vi "Write.vi"(10 "error in (no error)":errorcluster, 11 "Process_REF":string="Temperature") -> (0 "error out":errorcluster)   [LabVIEW 2018]
uses:
  <vilib>/DAQmx/write.llb/DAQmx Write (Digital Bool 1Line 1Point).vi
  <vilib>/DAQmx/create/channels.llb/DAQmx Create Channel (DO-Digital Output).vi
  <vilib>/DAQmx/miscellaneous.llb/DAQmx Fill In Error Info.vi
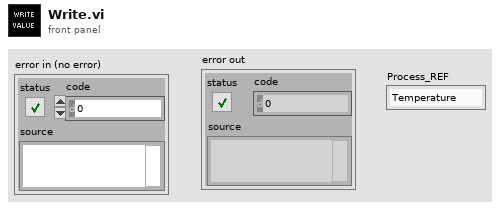
[diagram p1: front panel]
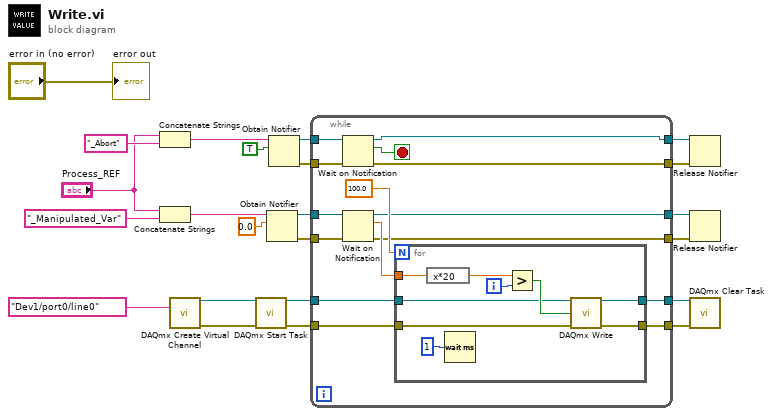
[diagram p0: block diagram]
diagram:
  n1 = Concatenate Strings("Process_REF", "_Abort" ("name (unnamed)")) -> (w1:string)
  n2 = Concatenate Strings("Process_REF", "_Manipulated_Var" ("name (unnamed)")) -> (w5:string)
  n3 = call-poly <vilib>:"DAQmx Create Virtual Channel.vi"("lines"=tag "Dev1/port0/line0") -> ("task out"=w23:refnum<k21>, "error out"=w22:errorcluster)  [unwired: 13 in]
  n4 = call <vilib>:"DAQmx Start Task.vi"("task/channels in"=w23, "error in"=w22) -> ("task out"=w20:refnum<k21>, "error out"=w19:errorcluster)  [unwired: 12 in]
  n5 = Obtain Notifier(name (unnamed)=w5, notification data type=0.0) -> (notifier out=w16:refnum<notifier>, error out=w14:errorcluster)  [unwired: 2 in, 1 out]
  n6 = Obtain Notifier(name (unnamed)=w1, notification data type=TRUE) -> (notifier out=w11:refnum<notifier>, error out=w10:errorcluster)  [unwired: 2 in, 1 out]
  n7 = while {
    tunnel: w20 -> [w27]
    tunnel: w19 -> [w24]
    tunnel: [w26] -> w18
    tunnel: [w25] -> w17
    tunnel: w16 -> [w36]
    tunnel: w14 -> [w35]
    tunnel: [w34] -> w13
    tunnel: [w33] -> w12
    tunnel: w11 -> [w32]
    tunnel: w10 -> [w31]
    tunnel: [w30] -> w9
    tunnel: [w29] -> w8
    stop <- w28 stop-if-true
    n8 = Wait on Notification(notifier=w32, error in (no error)=w31) -> (notifier out=w30:refnum<notifier>, notification=w28:bool, error out=w29:errorcluster)  [unwired: 2 in, 1 out]
    n9 = Wait on Notification(notifier=w36, error in (no error)=w35) -> (notifier out=w34:refnum<notifier>, notification=w37:dbl, error out=w33:errorcluster)  [unwired: 2 in, 1 out]
    n10 = for {
      N: 100.0 -> [_]
      tunnel: w37 -> [w45]
      tunnel: w27 -> [w42]
      tunnel: [w41] -> w26
      tunnel: [w40] -> w25
      tunnel: w24 -> [w39]
      i -> [w47]
      n11 = expression code="x*20"(w45) -> (w46:dbl)
      n12 = Wait (ms)(milliseconds to wait=u32 1) -> ()  [unwired: 1 out]
      n13 = Greater?(x=w46, y=w47) -> (0:w43:bool)
      n14 = call-poly <vilib>:"DAQmx Write.vi"("task/channels in"=w42, "data"=w43, "error in"=w39) -> ("task out"=w41:refnum<k21>, "error out"=w40:errorcluster)  [unwired: 10 in, 1 out]
    }
  }
  n15 = Release Notifier(notifier=w9, error in (no error)=w8) -> ()  [unwired: 1 in, 3 out]
  n16 = Release Notifier(notifier=w13, error in (no error)=w12) -> ()  [unwired: 1 in, 3 out]
  n17 = call <vilib>:"DAQmx Clear Task.vi"("task in"=w18, "error in"=w17) -> ()  [unwired: 13 in, 1 out]
  "error out" <- "error in (no error)"
